vi "Read.vi"(8 "error in (no error)":errorcluster, 11 "Add_WFM in":refnum<class "AbsFunc_One Term_WFM_Numeric.lvclass">) -> (0 "error out":errorcluster, 2 "Waveform":waveform(dbl), 3 "Add_WFM out":refnum<class "AbsFunc_One Term_WFM_Numeric.lvclass">)   [LabVIEW 2021, in "AbsFunc_One Term_WFM_Numeric.lvclass"]
uses:
  AbsFunc_One Term_WFM_Numeric.lvclass
  AbsFunc_One Term_WFM_Numeric.lvclass/AbsFunc_One Term_WFM_Numeric.ctl
  Abs_Types/Waveform/Abs_Waveform.lvclass
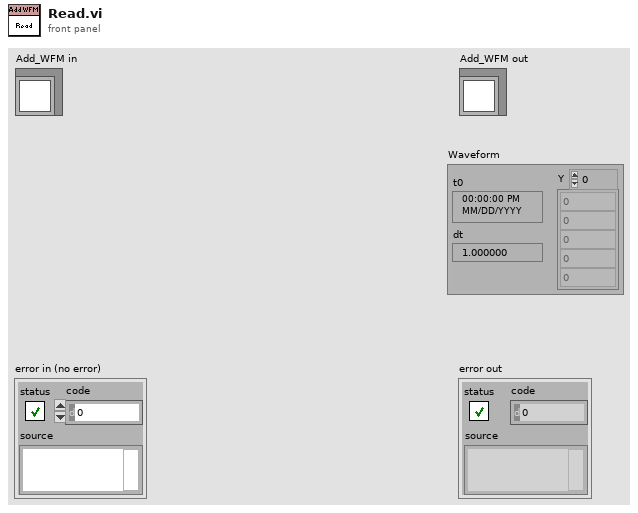
[diagram p1: front panel]
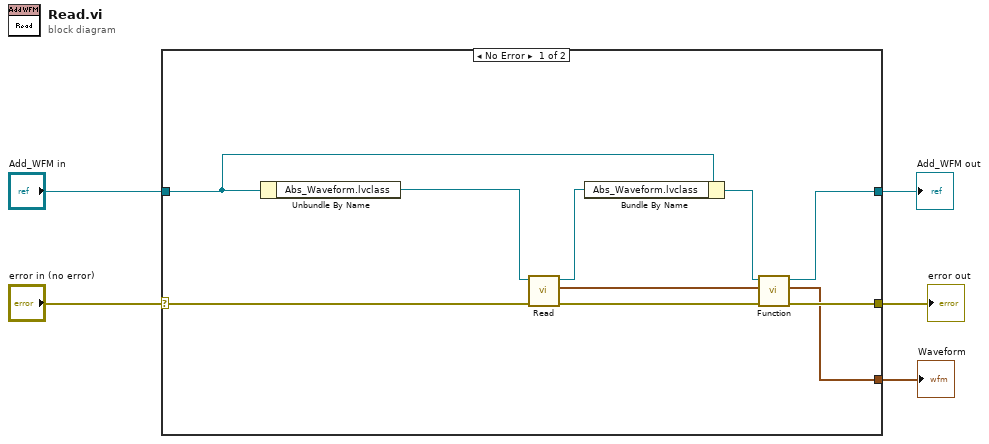
[diagram p0: block diagram]
diagram:
  n1 = case shown="No Error" "error in (no error)" {
    selector: "error in (no error)" -> [w14 w16]
    tunnel: [w15 w16] -> w5
    tunnel: [w12 w17] -> w4
    tunnel: "Add_WFM in" -> [w13 w17]
    tunnel: [w11 _] -> w1
    frame No Error {
      n2 = Unbundle By Name(w13) -> ("Abs_Waveform.lvclass"=w8:refnum<class "Abs_Waveform.lvclass">)
      n3 = call-dynamic "Read.vi"("error in (no error)"=w14, "Abs_Waveform in"=w8) -> ("error out"=w10:errorcluster, "Waveform"=w6:waveform(dbl), "Abs_Waveform out"=w7:refnum<class "Abs_Waveform.lvclass">)  [unwired: 7 in]
      n4 = Bundle By Name(cluster=w13, "Abs_Waveform.lvclass"=w7) -> (w9:refnum<class "AbsFunc_One Term_WFM_Numeric.lvclass">)
      n5 = call-dynamic "Function.vi"("error in (no error)"=w10, "Waveform"=w6, "Two Terminal in"=w9) -> ("error out"=w15:errorcluster, "Result"=w11:waveform(dbl), "Two Terminal out"=w12:refnum<class "AbsFunc_One Term_WFM_Numeric.lvclass">)  [unwired: 6 in]
    }
    frame Error {
    }
  }
  "error out" <- w5
  "Add_WFM out" <- w4
  "Waveform" <- w1
